vi "Simulated_Field_Prepare_PNG.vi"(11 "path to PNG file":path) -> (2 "new picture":picture, 3 "Draw Area Size":T1)   [LabVIEW 2019, in "Simulated_Field.lvlib"]
uses:
  <vilib>/Utility/miscctls.llb/LVBoundsTypeDef.ctl
  Simulated_Field.lvlib
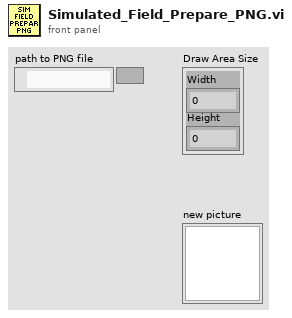
[diagram p1: front panel]
types:
  T1 = typedef "LVBoundsTypeDef.ctl" = cluster{"Width":u32, "Height":u32}
  T2 = typedef "imagedata.ctl" = cluster{"image type":i32, "image depth":i32, "image":u8[], "mask":u8[], "colors":u32[], "Rectangle":cluster{"left":i16, "top":i16, "right":i16, "bottom":i16}}
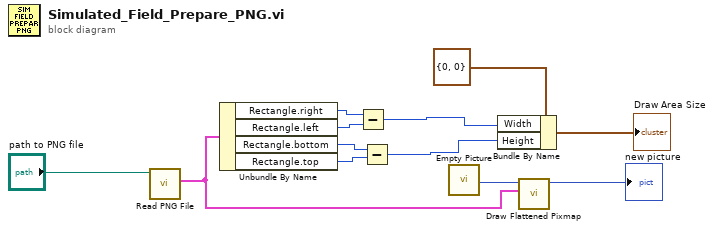
[diagram p0: block diagram]
diagram:
  n1 = call <vilib>:"Read PNG File.vi"("path to PNG file"="path to PNG file") -> ("image data"=w2:T2)  [unwired: 8 in, 2 out]
  n2 = Unbundle By Name(w2) -> ("Rectangle.right"=w7:i16, "Rectangle.left"=w6:i16, "Rectangle.bottom"=w8:i16, "Rectangle.top"=w5:i16)
  n3 = Subtract(x=w7, y=w6) -> (x-y=w11:i16)
  n4 = Subtract(x=w8, y=w5) -> (x-y=w12:i16)
  n5 = call "Empty Picture"() -> ("empty picture"=w3:picture)
  n6 = Bundle By Name(cluster=T1 {"Width"=0, "Height"=0} ("Draw Area Size"), "Width"=w11, "Height"=w12) -> (→"Draw Area Size":T1)
  n7 = call <vilib>:"Draw Flattened Pixmap.vi"("image data"=w2, "picture"=w3) -> ("new picture"=→"new picture":picture)  [unwired: 7 in]
